vi "Untitled 2.vi"() -> ()   [LabVIEW 2014]
panel:
  out "error out 2":errorcluster
  out "Numeric":i32
  out "data out 2":string
  out "?":bool
  out "array":bool[](array[boolean])
  out "error out":errorcluster
  out "data out":string
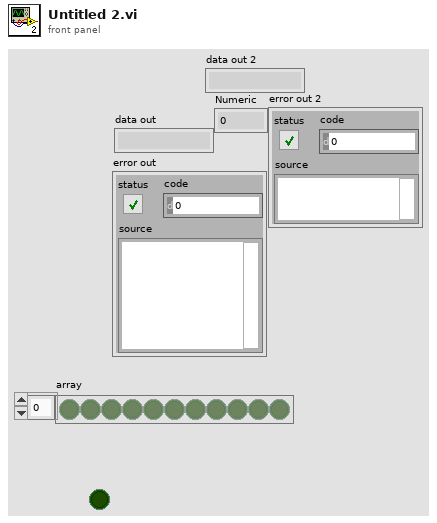
[diagram p1: front panel]
types:
  T1 = enum16{"Standard", "Buffered", "CRLF", "Immediate"}
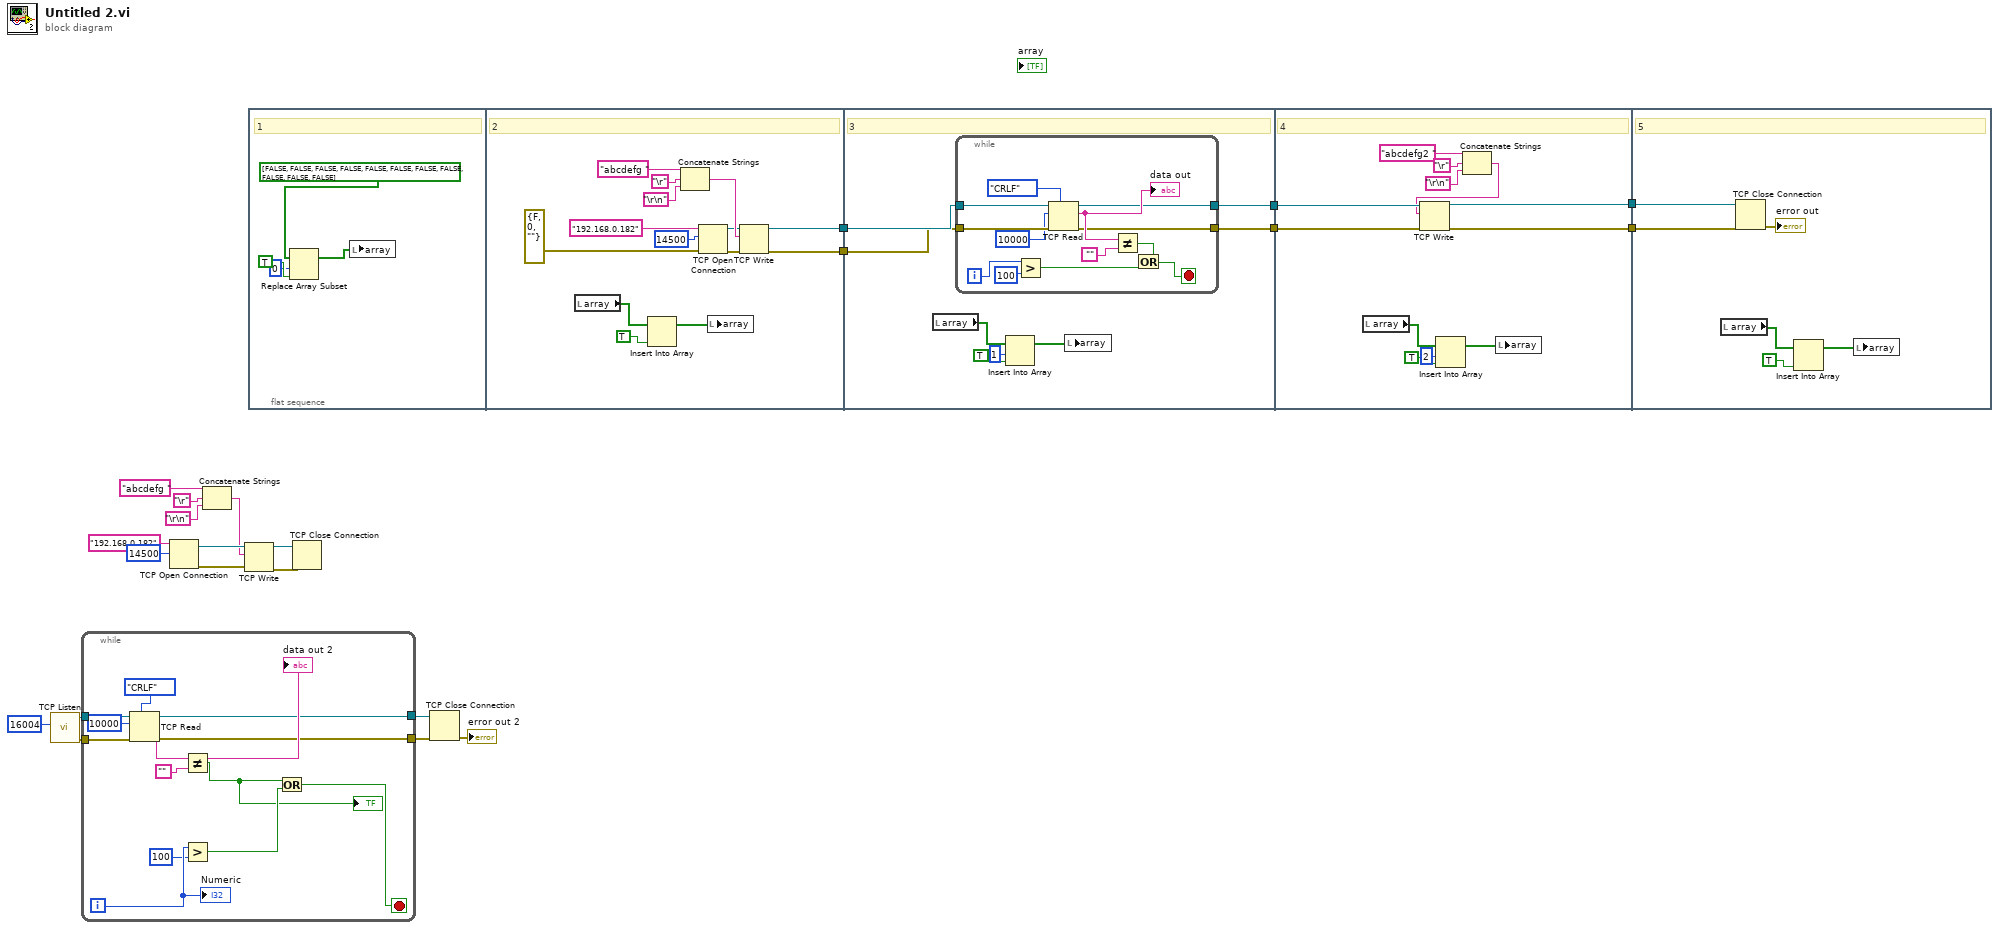
[diagram p0: block diagram]
diagram:
  n1 = call <vilib>:"TCP Listen.vi"("port"=u16 16004) -> ("error out"=w20:errorcluster, "connection ID"=w21:refnum<k5>)  [unwired: 6 in, 3 out]
  n2 = while {
    tunnel: w21 -> [w34]
    tunnel: w20 -> [w35]
    tunnel: [w26] -> w18
    tunnel: [w25] -> w19
    i -> [w29]
    stop <- w24 stop-if-true
    n3 = TCP Read(connection ID=w34, bytes to read=10000, error in (no error)=w35, 7:T1."CRLF" ("mode (standard)")) -> (connection ID out=w26:refnum<k5>, data out=w31:string, error out=w25:errorcluster)  [unwired: 1 in]
    "data out 2" <- w31
    n4 = Not Equal?(x=w31, y="") -> (x != y?=w23:bool)
    "?" <- w23
    n5 = Greater?(x=w29, y=100) -> (0:w27:bool)
    n6 = Or(x=w23, y=w27) -> (x .or. y?=w24:bool)
    "Numeric" <- w29
  }
  n7 = TCP Open Connection(address="192.168.0.182", remote port or service name=u16 14500) -> (connection ID=w8:refnum<k5>, error out=w7:errorcluster)  [unwired: 3 in]
  n8 = Concatenate Strings("abcdefg ", "\r", "\r\n") -> (w3:string)
  n9 = TCP Write(connection ID=w8, data in=w3, error in (no error)=w7) -> (connection ID out=w1:refnum<k5>, error out=w2:errorcluster)  [unwired: 1 in, 1 out]
  n10 = flat-sequence {
    tunnel: [w45] -> w16
    tunnel: [w44] -> w15
    tunnel: w16 -> [w61]
    tunnel: w15 -> [w60]
    tunnel: [w59] -> w14
    tunnel: [w58] -> w13
    tunnel: w14 -> [w86]
    tunnel: w13 -> [w85]
    tunnel: [w80] -> w12
    tunnel: [w79] -> w11
    tunnel: w12 -> [w91]
    tunnel: w11 -> [w90]
    frame #0 {
      # "1"
      n11 = Replace Array Subset(array=bool[] [FALSE, FALSE, FALSE, FALSE, FALSE, FALSE, FALSE, FALSE, FALSE, FALSE, FALSE], new element=TRUE, index=0) -> (w39:bool[])
      n12 = local write "array"(w39) -> ()
    }
    frame #1 {
      # "2"
      n13 = local read "array"() -> (w41:bool[])
      n14 = Insert Into Array(array=w41, new element=TRUE) -> (w42:bool[])  [unwired: 1 in]
      n15 = Concatenate Strings("abcdefg ", "\r", "\r\n") -> (w53:string)
      n16 = TCP Open Connection(address="192.168.0.182", remote port or service name=u16 14500, error in (no error)=errorcluster {"status"=FALSE, "code"=0, "source"=""}) -> (connection ID=w48:refnum<k5>, error out=w49:errorcluster)  [unwired: 2 in]
      n17 = local write "array"(w42) -> ()
      n18 = TCP Write(connection ID=w48, data in=w53, error in (no error)=w49) -> (connection ID out=w45:refnum<k5>, error out=w44:errorcluster)  [unwired: 1 in, 1 out]
    }
    frame #2 {
      # "3"
      n19 = local read "array"() -> (w57:bool[])
      n20 = while {
        tunnel: w61 -> [w74]
        tunnel: w60 -> [w73]
        tunnel: [w68] -> w58
        tunnel: [w62] -> w59
        i -> [w65]
        stop <- w70 stop-if-true
        n21 = Greater?(x=w65, y=100) -> (0:w63:bool)
        n22 = TCP Read(connection ID=w74, bytes to read=10000, error in (no error)=w73, 7:T1."CRLF" ("mode (standard)")) -> (connection ID out=w62:refnum<k5>, data out=w72:string, error out=w68:errorcluster)  [unwired: 1 in]
        "data out" <- w72
        n23 = Not Equal?(x=w72, y="") -> (x != y?=w69:bool)
        n24 = Or(x=w69, y=w63) -> (x .or. y?=w70:bool)
      }
      n25 = Insert Into Array(array=w57, index=1, new element=TRUE) -> (w56:bool[])
      n26 = local write "array"(w56) -> ()
    }
    frame #3 {
      # "4"
      n27 = local read "array"() -> (w76:bool[])
      n28 = Insert Into Array(array=w76, index=2, new element=TRUE) -> (w77:bool[])
      n29 = Concatenate Strings("abcdefg2 ", "\r", "\r\n") -> (w81:string)
      n30 = TCP Write(connection ID=w86, data in=w81, error in (no error)=w85) -> (connection ID out=w80:refnum<k5>, error out=w79:errorcluster)  [unwired: 1 in, 1 out]
      n31 = local write "array"(w77) -> ()
    }
    frame #4 {
      # "5"
      n32 = local read "array"() -> (w89:bool[])
      n33 = TCP Close Connection(connection ID=w91, error in (no error)=w90) -> (error out=→"error out":errorcluster)  [unwired: 1 in, 1 out]
      n34 = Insert Into Array(array=w89, new element=TRUE) -> (w88:bool[])  [unwired: 1 in]
      n35 = local write "array"(w88) -> ()
    }
  }
  n36 = TCP Close Connection(connection ID=w1, error in (no error)=w2) -> ()  [unwired: 1 in, 2 out]
  n37 = TCP Close Connection(connection ID=w18, error in (no error)=w19) -> (error out=→"error out 2":errorcluster)  [unwired: 1 in, 1 out]
